vi "ReadData3.vi"() -> ()   [LabVIEW 2013]
uses:
  <vilib>/Utility/file.llb/Read From Spreadsheet File (DBL).vi
  <vilib>/Analysis/NI_AALPro.lvlib
panel:
  out "Fmin":dbl format="%#_13g"
  out "Fmax":dbl format="%#_13g"
  out "# Data points":i32
  out "Peak Area (V-MHz)":dbl=0.0044393014138011675 format="%#_3g"
  out "Linear Slope (V/MHz)":dbl=0.16224074589285484 format="%#_3g"
  out "RMS Fit Error (V)":dbl=0.01168943219151948 format="%#_2g"
  in  "Start sigma (V)":dbl=0.01 format="%#_13g"
  in  "Start offset (V)":dbl format="%#_13g"
  out "FWHM (MHz)":dbl=0.0069336117351933855 format="%#_3g"
  out "Center Freq (MHz)":dbl=224.7917277288786
  out "Amplitude (V)":dbl=0.25549081559976244 format="%#_3g"
  out "NMR Graph + Fit":cluster{cluster{dbl, "Numeric":dbl}[]}[](graph)
  out "File size (bytes)":i32=3882
  out "Waveform Array":dbl[](array[numeric])=[224.59, -0.0399079]
  out "File name":string="C:\\Documents and Settings\\Patrick McGaughey\\Desktop\\rssmt\\wfm.txt"
  # "Gaussian Fit Results"
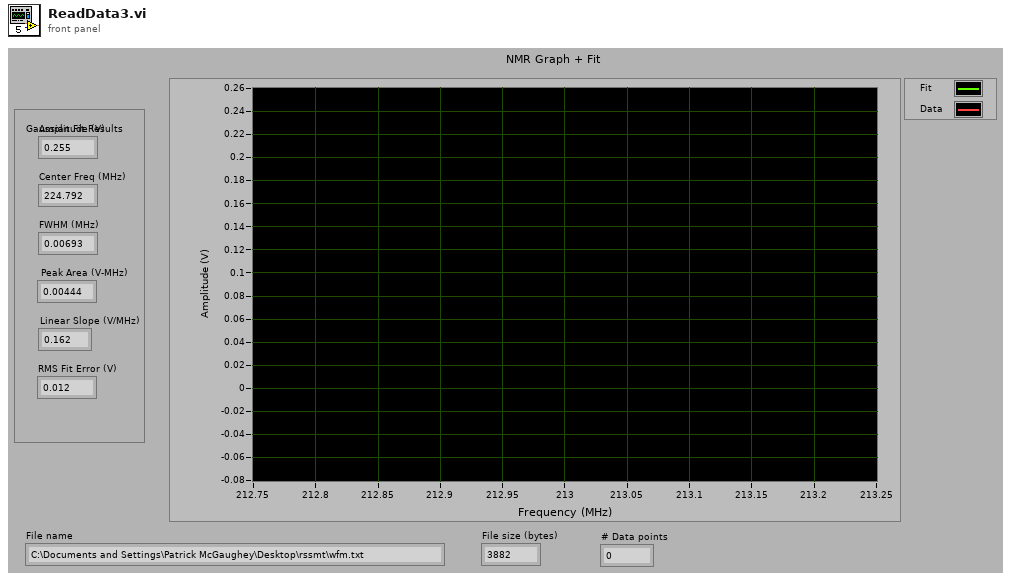
[diagram p1: front panel]
types:
  T1 = cluster{dbl, dbl, "Start sigma (V)":dbl, "Start offset (V)":dbl}
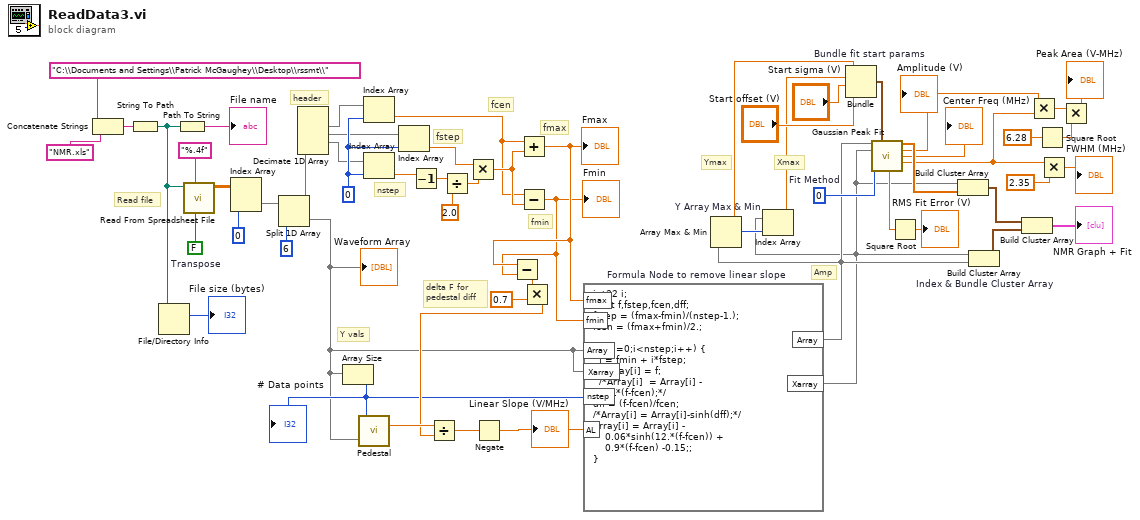
[diagram p0: block diagram]
diagram:
  w10 = 0
  w43 = 0  # Fit Method
  w54 = FALSE  # Transpose
  # "Read file"
  # "header"
  # "nstep"
  # "fstep"
  # "fcen"
  # "fmin"
  # "fmax"
  # "Amp"
  # "delta F for\npedestal diff"
  # "Ymax"
  # "Xmax"
  # "Y vals"
  n1 = Concatenate Strings "Concatenate Strings"("C:\\Documents and Settings\\Patrick McGaughey\\Desktop\\rssmt\\", "NMR.xls") -> (w57:string)
  n2 = String To Path(string=w57) -> (path=w53:path)
  n3 = File/Directory Info(path=w53) -> (size=→"File size (bytes)":i64)  [unwired: 1 in, 6 out]
  n4 = Path To String(path=w53) -> (string=→"File name":string)
  n5 = call-poly <vilib>:"Read From Spreadsheet File.vi"("transpose (no:F)"=w54, "format (%.3f)"="%.4f", "file path (dialog if empty)"=w53) -> ("all rows"=w19:dbl[][])  [unwired: 4 in, 4 out]
  n6 = Index Array "Index Array"(array=w19, index (col)=0) -> (element=w17:dbl[])  [unwired: 1 in]
  n7 = Split 1D Array(array=w17, index=6) -> (first subarray=w20:dbl[], second subarray=w2:dbl[])
  "Waveform Array" <- w2
  n8 = Decimate 1D Array(w20) -> (w12:dbl[], w9:dbl[], w8:dbl[])  [unwired: 3 out]
  n9 = Array Size(array=w2) -> (size(s)=w22:i32)
  "# Data points" <- w22
  n10 = call "Pedestal.vi"("Varray"=w2, "ArraySize"=w22) -> ("L-R"=w35:dbl)  [unwired: 1 out]
  n11 = Index Array "Index Array"(array=w12, index=w10) -> (element=w11:dbl)
  n12 = Index Array(array=w8, index=w10) -> (element=w6:dbl)
  n13 = Index Array(array=w9, index=w10) -> (element=w7:dbl)
  n14 = Decrement(x=w6) -> (x-1=w16:dbl)
  n15 = Divide(x=w16, y=2.0) -> (x/y=w14:dbl)
  n16 = Multiply(x=w7, y=w14) -> (x*y=w13:dbl)
  n17 = Add(x=w11, y=w13) -> (x+y=w4:dbl)
  "Fmax" <- w4
  n18 = Subtract(x=w11, y=w13) -> (x-y=w3:dbl)
  "Fmin" <- w3
  n19 = Subtract(x=w4, y=w3) -> (x-y=w33:dbl)
  n20 = Multiply(x=w33, y=0.7) -> (x*y=w32:dbl)
  n21 = Divide(x=w35, y=w32) -> (x/y=w31:dbl)
  n22 = Negate(x=w31) -> (-x=w5:dbl)
  "Linear Slope (V/MHz)" <- w5
  n23 = formula code="int32 i;\nfloat f,fstep,fcen,dff;\nfstep = (fmax-fmin)/(nstep-1.);\nfcen = (fmax+fmin)/2.;\n\nfor (i=0;i<nstep;i++) {\n  f = fmin + i*fstep;\n  Xarray[i] = f;\n  /*Array[i]  = Array[i] - \n    AL*(f-fcen);*/\ndff = (f-fcen)/fcen;\n/*Array[i] = Array[i]-sinh(dff);*/\nArray[i] = Array[i] - \n    0.06*sinh(12.*(f-fcen)) +\n    0.9*(f-fcen) -0.15;;\n}" "Formula Node to remove linear slope"("nstep"=w22, "fmin"=w3, "fmax"=w4, "AL"=w5, "Array"=w2, "Xarray"=w2) -> ("Array"=w24:dbl[], "Xarray"=w23:dbl[])
  n24 = Array Max & Min "Y Array Max & Min"(array=w24) -> (max value=w42:dbl, max index (indices)=w41:i32)  [unwired: 2 out]
  n25 = Index Array "Index Array"(array=w23, index=w41) -> (element=w28:dbl)
  n26 = Bundle "Bundle fit start params"(w42, w28, "Start sigma (V)"="Start sigma (V)", "Start offset (V)"="Start offset (V)") -> (w48:T1)  [unwired: 1 in]
  n27 = call <vilib>:"Gaussian Peak Fit.vi"("Y"=w24, "initial guess"=w48, "X"=w23, "method"=w43) -> ("Best Gaussian Fit"=w51:dbl[], "amplitude"=w40:dbl, "center"=→"Center Freq (MHz)":dbl, "standard deviation"=w27:dbl, "residue"=w30:dbl)  [unwired: 5 in, 2 out]
  "Amplitude (V)" <- w40
  n28 = Square Root(x=w30) -> (sqrt(x)=→"RMS Fit Error (V)":dbl)
  n29 = Build Cluster Array ("Index & Bundle Cluster Array")(w23, w51) -> (w1:cluster{dbl, "Numeric":dbl}[])
  n30 = Build Cluster Array "Index & Bundle Cluster Array"(w23, w24) -> (w47:cluster{dbl, dbl}[])
  n31 = Build Cluster Array "Build Cluster Array"(w1, w47) -> (→"NMR Graph + Fit":cluster{cluster{dbl, "Numeric":dbl}[]}[])
  n32 = Multiply(x=w40, y=w27) -> (x*y=w37:dbl)
  n33 = Square Root(x=6.28) -> (sqrt(x)=w38:dbl)
  n34 = Multiply(x=w27, y=2.35) -> (x*y=→"FWHM (MHz)":dbl)
  n35 = Multiply(x=w37, y=w38) -> (x*y=→"Peak Area (V-MHz)":dbl)
